vi "EtherNet CIP Read_core.vi"(0 "Connection Cluster in":T1, 1 "Tag":string, 4 "No of Elements":u8=1, 7 "error in (no error)":errorcluster) -> (14 "BOOL":bool, 15 "CONTROL/TIMER/COUNTER":T2, 16 "BOOL Array":bool[](array[boolean]), 17 "REAL Array":sgl[](array[numeric]), 20 "Connection Cluster out":T1, 21 "SINT Array":u8[](array[numeric]), 22 "INT Array":u16[](array[numeric]), 23 "DINT Array":u32[](array[numeric]), 26 "Datatype":T3(ring), 27 "error out":errorcluster)   [LabVIEW 2012]
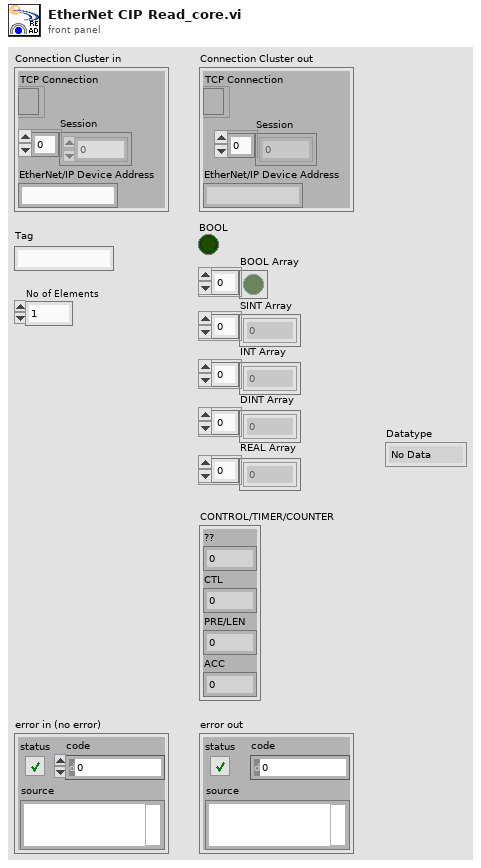
[diagram p1: front panel]
types:
  T1 = cluster{"TCP Connection":refnum<k5>, "Session":u8[], "EtherNet/IP Device Address":string}
  T2 = cluster{"??":u16, "CTL":u32, "PRE/LEN":u32, "ACC":u32}
  T3 = enum16{"No Data", "BOOL", "BIT Array", "SINT", "INT", "DINT", "REAL", "TIMER/CONTROL/COUNTER"}
  T4 = enum16{"Standard", "Buffered", "CRLF", "Immediate"}
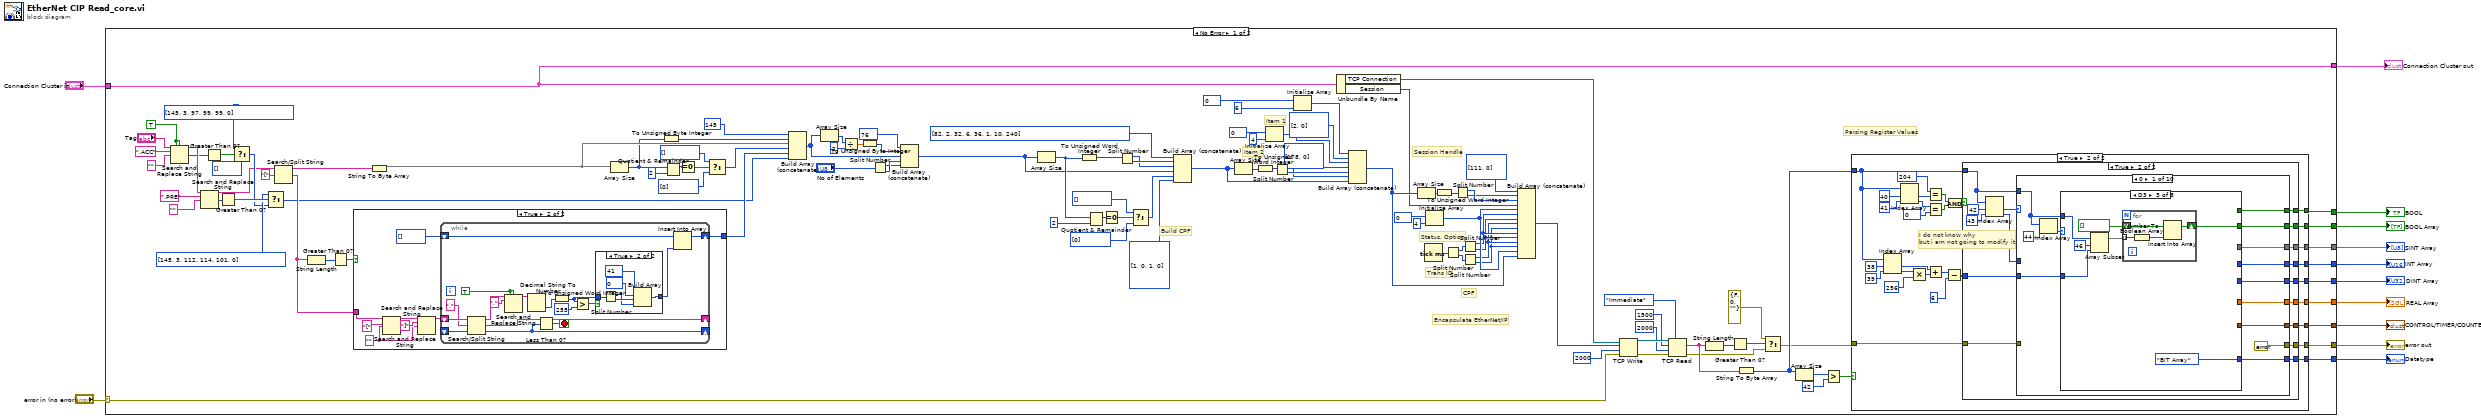
[diagram p0: block diagram]
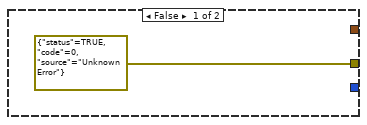
[diagram p3: hidden frame]
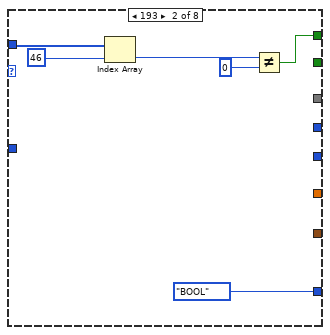
[diagram p5: hidden frame]
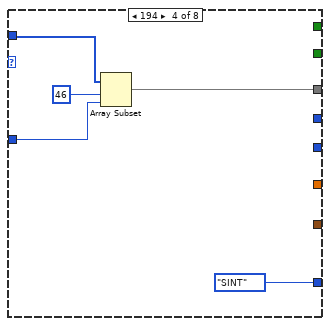
[diagram p6: hidden frame]
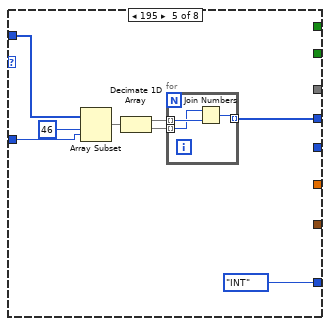
[diagram p7: hidden frame]
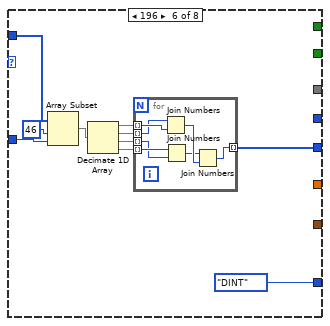
[diagram p8: hidden frame]
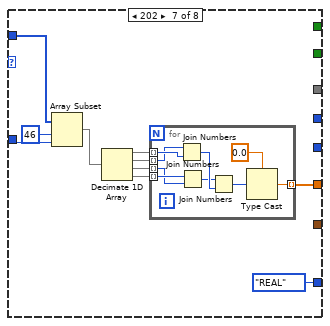
[diagram p9: hidden frame]
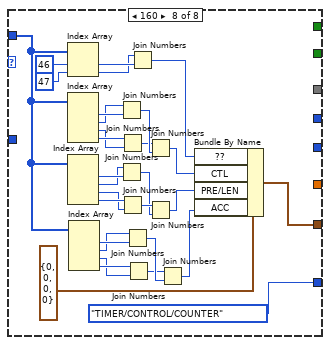
[diagram p10: hidden frame]
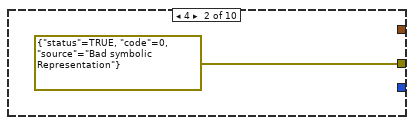
[diagram p11: hidden frame]
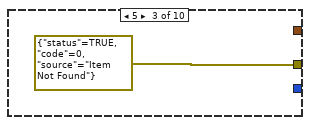
[diagram p12: hidden frame]
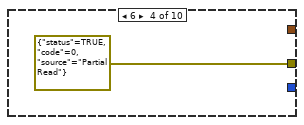
[diagram p13: hidden frame]
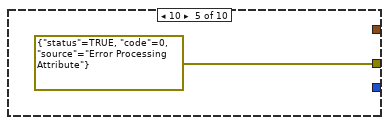
[diagram p14: hidden frame]
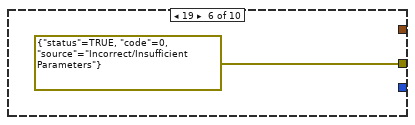
[diagram p15: hidden frame]
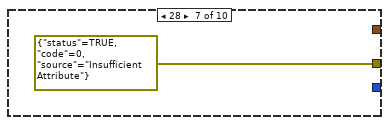
[diagram p16: hidden frame]
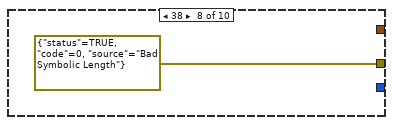
[diagram p17: hidden frame]
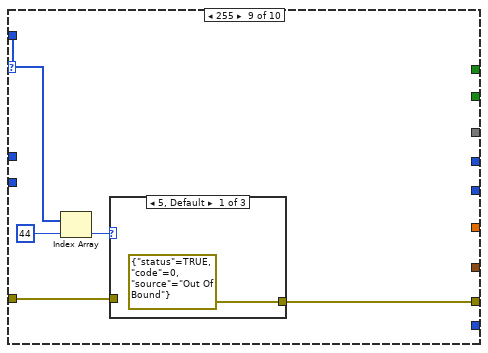
[diagram p18: hidden frame]
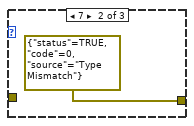
[diagram p19: hidden frame]
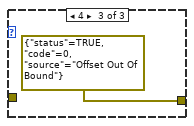
[diagram p20: hidden frame]
diagram:
  n1 = case shown="No Error" "error in (no error)" {
    selector: "error in (no error)" -> [w19 _]
    tunnel: "Connection Cluster in" -> [w126 w339]
    tunnel: [w126 w339] -> w9
    tunnel: [w31 _] -> w1
    tunnel: [w30 _] -> w12
    tunnel: [w29 _] -> w2
    tunnel: [w28 _] -> w3
    tunnel: [w27 _] -> w4
    tunnel: [w26 _] -> w5
    tunnel: [w25 _] -> w6
    tunnel: [w24 _] -> w10
    tunnel: [w21 errorcluster {"status"=TRUE, "code"=0, "source"="Unknown Error"} ("error out 2")] -> w11
    frame No Error {
      w81 = TRUE ("replace all? (F)")
      # "Parsing Register Values"
      # "Build CPF"
      # "Trans ID"
      # "CPF"
      # "Status, Option"
      # "Session Handle"
      # "Item 2"
      # "Item 1"
      # "Encapsulate EtherNet/IP"
      n2 = Search and Replace String(replace all?=w81, case sensitive?=w81, input string="Tag", search string=".ACC", replace string="" ("replace string (\"\")")) -> (result string=w78:string, number of replacements=w77:i32)  [unwired: 3 in, 2 out]
      n3 = Search and Replace String(input string=w78, search string=".PRE", replace string="" ("replace string (\"\")")) -> (result string=w68:string, number of replacements=w76:i32)  [unwired: 5 in, 2 out]
      n4 = Greater Than 0?(x=w77) -> (x > 0?=w75:bool)
      n5 = Greater Than 0?(x=w76) -> (x > 0?=w74:bool)
      n6 = Select(t=u8[] [145, 3, 97, 99, 99, 0], s=w75, f=u8[] []) -> (s? t:f=w71:u8[])
      n7 = Select(t=u8[] [145, 3, 112, 114, 101, 0], s=w74, f=w71) -> (s? t:f=w20:u8[])
      n8 = Search/Split String(string=w68, search string/char (-)="[") -> (substring before match=w67:string, match + rest of string=w48:string)  [unwired: 1 in, 1 out]
      n9 = String Length(string=w48) -> (length=w50:i32)
      n10 = Greater Than 0?(x=w50) -> (x > 0?=w49:bool)
      n11 = case shown="True" w49 {
        tunnel: w48 -> [_ w304]
        tunnel: [u8[] [] w303] -> w47
        frame False {
        }
        frame True {
          w307 = "" ("replace string (\"\")")
          n12 = Search and Replace String(input string=w304, search string="[", replace string=w307) -> (result string=w309:string)  [unwired: 5 in, 3 out]
          n13 = Search and Replace String(input string=w309, search string="]", replace string=w307) -> (result string=w306:string)  [unwired: 5 in, 3 out]
          n14 = while {
            shift-right: [w320] -> _
            shift-left: _ -> [w327]
            shift-right: [w325] -> _
            shift-left: w306 -> [w326]
            shift-right: [w312] -> w303
            shift-left: u8[] [] -> [w314]
            stop <- w321 stop-if-true
            w319 = TRUE ("replace all? (F)")
            n15 = Search/Split String(string=w326, search string/char (-)=",", offset (0)=w327) -> (substring before match=w323:string, match + rest of string=w325:string, offset of match=w320:i32)
            n16 = Search and Replace String(replace all?=w319, case sensitive?=w319, input string=w323, search string=",") -> (result string=w318:string)  [unwired: 4 in, 3 out]
            n17 = Decimal String To Number(string=w318) -> (number=w315:i32)  [unwired: 2 in, 1 out]
            n18 = Less Than 0?(x=w320) -> (x < 0?=w321:bool)
            n19 = To Unsigned Word Integer(number=w315) -> (unsigned 16bit integer=w311:u16)
            n20 = Greater?(x=w311, y=u16 255) -> (0:w316:bool)
            n21 = case shown="True" w316 {
              tunnel: w311 -> [w331 w337]
              tunnel: [w328 w332] -> w313
              frame False {
                n22 = To Unsigned Byte Integer(number=w331) -> (unsigned 8bit integer=w330:u8)
                n23 = Build Array(u8 40 ("Status"), w330) -> (w328:u8[])
              }
              frame True {
                n24 = Split Number(x=w337) -> (hi(x)=w335:u8, lo(x)=w336:u8)
                n25 = Build Array(u8 41 ("Status"), u8 0 ("Status"), w336, w335) -> (w332:u8[])
              }
            }
            n26 = Insert Into Array(array=w314, new element=w313) -> (w312:u8[])  [unwired: 1 in]
          }
        }
      }
      n27 = String To Byte Array(string=w67) -> (unsigned byte array=w65:u8[])
      n28 = Array Size(array=w65) -> (size(s)=w52:i32)
      n29 = To Unsigned Byte Integer(number=w52) -> (unsigned 8bit integer=w64:u8)
      n30 = Quotient & Remainder(x=w52, y=2) -> (x-y*floor(x/y)=w54:i32)  [unwired: 1 out]
      n31 = Equal To 0?(x=w54) -> (x = 0?=w57:bool)
      n32 = Select(t=u8[] [], s=w57, f=u8[] [0]) -> (s? t:f=w51:u8[])
      n33 = Build Array (concatenate)(u8 145 ("Status"), w64, w65, w51, w47, w20) -> (w41:u8[])
      n34 = Array Size(array=w41) -> (size(s)=w44:i32)
      n35 = Divide(x=w44, y=u8 2) -> (x/y=w43:dbl)
      n36 = To Unsigned Byte Integer(number=w43) -> (unsigned 8bit integer=w42:u8)
      n37 = Split Number(x="No of Elements") -> (hi(x)=w38:u8, lo(x)=w39:u8)
      n38 = Build Array (concatenate)(u8 76 ("Status"), w42, w41, w39, w38) -> (w40:u8[])
      n39 = Array Size(array=w40) -> (size(s)=w58:i32)
      n40 = To Unsigned Word Integer(number=w58) -> (unsigned 16bit integer=w122:u16)
      n41 = Quotient & Remainder(x=w58, y=2) -> (x-y*floor(x/y)=w85:i32)  [unwired: 1 out]
      n42 = Equal To 0?(x=w85) -> (x = 0?=w60:bool)
      n43 = Split Number(x=w122) -> (hi(x)=w120:u8, lo(x)=w121:u8)
      n44 = Select(t=u8[] [], s=w60, f=u8[] [0]) -> (s? t:f=w59:u8[])
      n45 = Build Array (concatenate)(u8[] [82, 2, 32, 6, 36, 1, 10, 240], w121, w120, w40, w59, u8[] [1, 0, 1, 0]) -> (w87:u8[])
      n46 = Array Size(array=w87) -> (size(s)=w91:i32)
      n47 = To Unsigned Word Integer(number=w91) -> (unsigned 16bit integer=w92:u16)
      n48 = Initialize Array(u8 0 ("Status"), 4 ("dimension size")) -> (w89:u8[])
      n49 = Split Number(x=w92) -> (hi(x)=w88:u8, lo(x)=w90:u8)
      n50 = Initialize Array(u8 0 ("Status"), 6 ("dimension size")) -> (w18:u8[])
      n51 = Unbundle By Name(w126) -> ("TCP Connection"=w16:refnum<k5>, "Session"=w15:u8[])
      n52 = Build Array (concatenate)(w18, u8[] [2, 0], w89, u8[] [178, 0], w90, w88, w87) -> (w37:u8[])
      n53 = Array Size(array=w37) -> (size(s)=w116:i32)
      n54 = Tick Count (ms)() -> (millisecond timer value=w110:u32)
      n55 = Initialize Array(u8 0 ("Status"), 4 ("dimension size")) -> (w111:u8[])
      n56 = To Unsigned Word Integer(number=w116) -> (unsigned 16bit integer=w117:u16)
      n57 = Split Number(x=w110) -> (hi(x)=w109:u16, lo(x)=w108:u16)
      n58 = Split Number(x=w117) -> (hi(x)=w115:u8, lo(x)=w114:u8)
      n59 = Split Number(x=w109) -> (hi(x)=w107:u8, lo(x)=w106:u8)
      n60 = Split Number(x=w108) -> (hi(x)=w105:u8, lo(x)=w104:u8)
      n61 = Build Array (concatenate)(u8[] [111, 0], w114, w115, w15, w111, w107, w106, w105, w104, w107, w106, w105, w104, w111, w37) -> (w103:u8[])
      n62 = TCP Write(connection ID=w16, data in=w103, error in (no error)=w19, 9:2000 ("timeout ms (25000)")) -> (connection ID out=w124:refnum<k5>, error out=w125:errorcluster)  [unwired: 1 out]
      n63 = TCP Read(connection ID=w124, bytes to read=1500, error in (no error)=w125, 7:T4."Immediate" ("mode (standard)"), 9:2000 ("timeout ms (25000)")) -> (data out=w99:string, error out=w14:errorcluster)  [unwired: 1 out]
      n64 = String Length(string=w99) -> (length=w101:i32)
      n65 = Greater Than 0?(x=w101) -> (x > 0?=w100:bool)
      n66 = String To Byte Array(string=w99) -> (unsigned byte array=w32:u8[])
      n67 = Select(t=errorcluster {"status"=FALSE, "code"=0, "source"=""}, s=w100, f=w14) -> (s? t:f=w22:errorcluster)
      n68 = Array Size(array=w32) -> (size(s)=w35:i32)
      n69 = Greater?(x=w35, y=42) -> (0:w33:bool)
      n70 = case shown="True" w33 {
        tunnel: w32 -> [_ w139]
        tunnel: [_ w147] -> w31
        tunnel: [_ w146] -> w30
        tunnel: [_ w145] -> w29
        tunnel: [_ w144] -> w28
        tunnel: [_ w143] -> w27
        tunnel: [_ w142] -> w26
        tunnel: [_ w141] -> w25
        tunnel: [_ w140] -> w24
        tunnel: w22 -> [w127 w129]
        tunnel: [w127 w128] -> w21
        frame False {
        }
        frame True {
          # "I do not know why\nbut i am not going to modify it"
          n71 = Index Array(array=w139, index #1=38 ("index"), index #2=39 ("index")) -> (element #1=w133:u8, element #2=w136:u8)
          n72 = Index Array(array=w139, index #1=40 ("index"), index #2=41 ("index")) -> (element #1=w153:u8, element #2=w154:u8)
          n73 = Multiply(x=w136, y=u16 256) -> (x*y=w134:u16)
          n74 = Equal?(x=u8 204 ("Status"), y=w153) -> (x = y?=w149:bool)
          n75 = Equal?(x=w154, y=u8 0 ("Status")) -> (x = y?=w150:bool)
          n76 = Add(x=w133, y=w134) -> (x+y=w132:u16)
          n77 = Subtract(x=w132, y=u16 6) -> (x-y=w130:u16)
          n78 = And(x=w149, y=w150) -> (x .and. y?=w148:bool)
          n79 = case shown="True" w148 {
            tunnel: w139 -> [_ w170]
            tunnel: [_ w169] -> w147
            tunnel: [_ w168] -> w146
            tunnel: [_ w167] -> w145
            tunnel: [_ w166] -> w144
            tunnel: [_ w165] -> w143
            tunnel: [_ w164] -> w142
            tunnel: [_ w163] -> w141
            tunnel: [_ w162] -> w140
            tunnel: w130 -> [_ w161]
            tunnel: w129 -> [_ w160]
            tunnel: [errorcluster {"status"=TRUE, "code"=0, "source"="Unknown Error"} ("error out 2") w159] -> w128
            frame False {
            }
            frame True {
              n80 = Index Array(array=w170, index #1=42 ("index"), index #2=43 ("index")) -> (element #1=w171:u8, element #2=w158:u8)
              n81 = case shown="0" w171 {
                tunnel: w158 -> [_ _ _ _ _ _ _ _ _ _]
                tunnel: w170 -> [w184 _ _ _ _ _ _ _ w297 _]
                tunnel: [w183 _ _ _ _ _ _ _ _ _] -> w169
                tunnel: [w182 _ _ _ _ _ _ _ _ _] -> w168
                tunnel: [w181 _ _ _ _ _ _ _ _ _] -> w167
                tunnel: [w180 _ _ _ _ _ _ _ _ _] -> w166
                tunnel: [w179 _ _ _ _ _ _ _ _ _] -> w165
                tunnel: [w178 _ _ _ _ _ _ _ _ _] -> w164
                tunnel: [w177 _ _ _ _ _ _ _ _ _] -> w163
                tunnel: [w176 _ _ _ _ _ _ _ _ _] -> w162
                tunnel: w161 -> [w175 _ _ _ _ _ _ _ _ _]
                tunnel: w160 -> [_ _ _ _ _ _ _ _ w294 _]
                tunnel: [errorcluster {"status"=FALSE, "code"=0, "source"=""} ("error out 2") errorcluster {"status"=TRUE, "code"=0, "source"="Bad symbolic Representation"} ("error out 2") errorcluster {"status"=TRUE, "code"=0, "source"="Item Not Found"} ("error out 2") errorcluster {"status"=TRUE, "code"=0, "source"="Partial Read"} ("error out 2") errorcluster {"status"=TRUE, "code"=0, "source"="Error Processing Attribute"} ("error out 2") errorcluster {"status"=TRUE, "code"=0, "source"="Incorrect/Insufficient Parameters"} ("error out 2") errorcluster {"status"=TRUE, "code"=0, "source"="Insufficient Attribute"} ("error out 2") errorcluster {"status"=TRUE, "code"=0, "source"="Bad Symbolic Length"} ("error out 2") w293 errorcluster {"status"=TRUE, "code"=0, "source"="Unknown Error"} ("error out 2")] -> w159
                frame 0 {
                  n82 = Index Array(array=w184, index=44) -> (element=w185:u8)
                  n83 = case shown="D3" w185 {
                    tunnel: w184 -> [_ w192 w196 w207 w214 w223 w238 w281]
                    tunnel: [_ w188 _ _ _ _ _ _] -> w183
                    tunnel: [_ T3."BOOL" ("Datatype") T3."BIT Array" ("Datatype") T3."SINT" ("Datatype") T3."INT" ("Datatype") T3."DINT" ("Datatype") T3."REAL" ("Datatype") T3."TIMER/CONTROL/COUNTER" ("Datatype")] -> w182
                    tunnel: [_ _ w193 _ _ _ _ _] -> w181
                    tunnel: [_ _ _ w204 _ _ _ _] -> w180
                    tunnel: [_ _ _ _ w209 _ _ _] -> w179
                    tunnel: [_ _ _ _ _ w220 _ _] -> w178
                    tunnel: [_ _ _ _ _ _ w237 _] -> w177
                    tunnel: [_ _ _ _ _ _ _ w259] -> w176
                    tunnel: w175 -> [_ _ w197 w205 w213 w224 w239 _]
                    frame 0, Default {
                    }
                    frame 193 {
                      n84 = Index Array(array=w192, index=46) -> (element=w190:u8)
                      n85 = Not Equal?(x=w190, y=u8 0) -> (x != y?=w188:bool)
                    }
                    frame 211 {
                      n86 = Array Subset(array=w196, index=46, length=w197) -> (w195:u8[])
                      n87 = for {
                        tunnel: w195 -> [w203] mode=indexing
                        shift-right: [w200] -> w193
                        shift-left: bool[] [] -> [w202]
                        n88 = Number To Boolean Array(number=w203) -> (Boolean array=w201:bool[])
                        n89 = Insert Into Array(array=w202, new element=w201) -> (w200:bool[])  [unwired: 1 in]
                      }
                    }
                    frame 194 {
                      n90 = Array Subset(array=w207, index=46, length=w205) -> (w204:u8[])
                    }
                    frame 195 {
                      n91 = Array Subset(array=w214, index=46, length=w213) -> (w212:u8[])
                      n92 = Decimate 1D Array(w212) -> (w211:u8[], w210:u8[])
                      n93 = for {
                        tunnel: w211 -> [w219] mode=indexing
                        tunnel: w210 -> [w218] mode=indexing
                        tunnel: [w217] -> w209 mode=indexing
                        n94 = Join Numbers(hi=w218, lo=w219) -> ((hi.lo)=w217:u16)
                      }
                    }
                    frame 196 {
                      n95 = Array Subset(array=w223, index=46, length=w224) -> (w227:u8[])
                      n96 = Decimate 1D Array(w227) -> (w226:u8[], w225:u8[], w222:u8[], w221:u8[])
                      n97 = for {
                        tunnel: w226 -> [w234] mode=indexing
                        tunnel: w225 -> [w233] mode=indexing
                        tunnel: w222 -> [w231] mode=indexing
                        tunnel: w221 -> [w232] mode=indexing
                        tunnel: [w230] -> w220 mode=indexing
                        n98 = Join Numbers(hi=w233, lo=w234) -> ((hi.lo)=w236:u16)
                        n99 = Join Numbers(hi=w232, lo=w231) -> ((hi.lo)=w235:u16)
                        n100 = Join Numbers(hi=w235, lo=w236) -> ((hi.lo)=w230:u32)
                      }
                    }
                    frame 202 {
                      n101 = Array Subset(array=w238, index=46, length=w239) -> (w244:u8[])
                      n102 = Decimate 1D Array(w244) -> (w243:u8[], w242:u8[], w241:u8[], w240:u8[])
                      n103 = for {
                        tunnel: w243 -> [w253] mode=indexing
                        tunnel: w242 -> [w252] mode=indexing
                        tunnel: w241 -> [w250] mode=indexing
                        tunnel: w240 -> [w251] mode=indexing
                        tunnel: [w247] -> w237 mode=indexing
                        n104 = Join Numbers(hi=w252, lo=w253) -> ((hi.lo)=w255:u16)
                        n105 = Join Numbers(hi=w251, lo=w250) -> ((hi.lo)=w254:u16)
                        n106 = Join Numbers(hi=w254, lo=w255) -> ((hi.lo)=w248:u32)
                        n107 = Type Cast(type=sgl 0.0, x=w248) -> (*(type *) &x=w247:sgl)
                      }
                    }
                    frame 160 {
                      n108 = Index Array(array=w281, index #1=46 ("index"), index #2=47 ("index")) -> (element #1=w284:u8, element #2=w283:u8)
                      n109 = Index Array(array=w281) -> (element #1=w278:u8, element #2=w277:u8, element #3=w275:u8, element #4=w276:u8)  [unwired: 4 in]
                      n110 = Index Array(array=w281) -> (element #1=w270:u8, element #2=w268:u8, element #3=w266:u8, element #4=w267:u8)  [unwired: 4 in]
                      n111 = Index Array(array=w281) -> (element #1=w269:u8, element #2=w264:u8, element #3=w263:u8, element #4=w265:u8)  [unwired: 4 in]
                      n112 = Join Numbers(hi=w277, lo=w278) -> ((hi.lo)=w280:u16)
                      n113 = Join Numbers(hi=w268, lo=w270) -> ((hi.lo)=w273:u16)
                      n114 = Join Numbers(hi=w276, lo=w275) -> ((hi.lo)=w279:u16)
                      n115 = Join Numbers(hi=w267, lo=w266) -> ((hi.lo)=w274:u16)
                      n116 = Join Numbers(hi=w264, lo=w269) -> ((hi.lo)=w272:u16)
                      n117 = Join Numbers(hi=w265, lo=w263) -> ((hi.lo)=w271:u16)
                      n118 = Join Numbers(hi=w283, lo=w284) -> ((hi.lo)=w262:u16)
                      n119 = Join Numbers(hi=w279, lo=w280) -> ((hi.lo)=w256:u32)
                      n120 = Join Numbers(hi=w274, lo=w273) -> ((hi.lo)=w257:u32)
                      n121 = Join Numbers(hi=w271, lo=w272) -> ((hi.lo)=w261:u32)
                      n122 = Bundle By Name(cluster=T2 {"??"=0, "CTL"=0, "PRE/LEN"=0, "ACC"=0} ("CONTROL/TIMER/COUNTER"), "??"=w262, "CTL"=w256, "PRE/LEN"=w257, "ACC"=w261) -> (w259:T2)
                    }
                  }
                }
                frame 4 {
                }
                frame 5 {
                }
                frame 6 {
                }
                frame 10 {
                }
                frame 19 {
                }
                frame 28 {
                }
                frame 38 {
                }
                frame 255 {
                  n123 = Index Array(array=w297, index=44) -> (element=w295:u8)
                  n124 = case shown="5, Default" w295 {
                    tunnel: w294 -> [_ _ _]
                    tunnel: [errorcluster {"status"=TRUE, "code"=0, "source"="Out Of Bound"} ("error out 2") errorcluster {"status"=TRUE, "code"=0, "source"="Type Mismatch"} ("error out 2") errorcluster {"status"=TRUE, "code"=0, "source"="Offset Out Of Bound"} ("error out 2")] -> w293
                    frame 5, Default {
                    }
                    frame 7 {
                    }
                    frame 4 {
                    }
                  }
                }
                frame 1, Default {
                }
              }
            }
          }
        }
      }
    }
    frame Error {
    }
  }
  "Datatype" <- w12
  "error out" <- w11
  "CONTROL/TIMER/COUNTER" <- w10
  "Connection Cluster out" <- w9
  "BOOL" <- w1
  "BOOL Array" <- w2
  "SINT Array" <- w3
  "INT Array" <- w4
  "DINT Array" <- w5
  "REAL Array" <- w6
